vi "Digital IO Express.vi"() -> ()   [LabVIEW 2020]
panel:
  out "DI Read":u8
  in  "Stop":bool
  in  "DO":u8
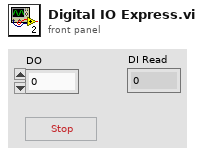
[diagram p1: front panel]
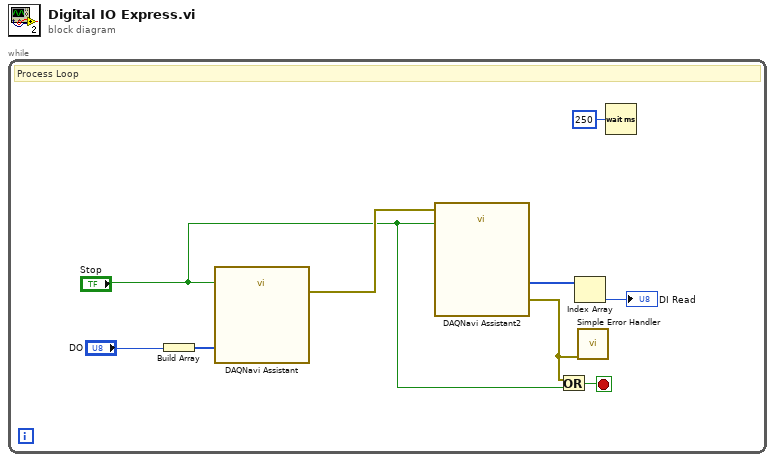
[diagram p0: block diagram]
diagram:
  n1 = while {
    stop <- w4 stop-if-true
    # "Process Loop"
    n2 = Build Array("DO") -> (w8:u8[])
    n3 = call "DAQNavi Assistant"("stop(true)"="Stop", "dataIn(U8Array)"=w8) -> ("error out"=w5:errorcluster)  [unwired: 25 in]
    n4 = call "DAQNavi Assistant2"("error in(no error)"=w5, "stop(true)"="Stop") -> ("error out"=w2:errorcluster, "dataOut(U8Array)"=w7:u8[])  [unwired: 24 in]
    n5 = Or(x=w2, y="Stop") -> (x .or. y?=w4:bool)
    n6 = Index Array(array=w7) -> (element=→"DI Read":u8)  [unwired: 1 in]
    n7 = call <vilib>:"Simple Error Handler.vi"("error in (no error)"=w2) -> ()  [unwired: 4 in, 5 out]
    n8 = Wait (ms)(milliseconds to wait=u32 250) -> ()  [unwired: 1 out]
  }
